vi "2012_01_03 Crunch.vi"(6 "Temp On":dbl, 7 "Motor #":i32, 8 "error in (no error)":errorcluster, 9 "data":waveform(dbl)[](array[waveform]), 10 "Elapsed Time (h)":dbl, 11 "Motor In":T1 {"Elec Power In (W)" format="%.3g"; "Efficiency" format="%#_3g%%"; "Mech Pwr Out (W)" format="%.3g"; "Torque (mNm)" format="%.3g"; "Elapsed Time (h)" format="%.1f"; "Supply (V)" format="%.2f"; "RPM" scale=0.0..40000.0 scale format="%#_4p"}) -> (0 "error out":errorcluster, 2 "Dynamic Data Type":dynamicdata(waveform), 3 "Motor Out":T1={"Enabled"=FALSE, "Fail"=FALSE, "RPM"=0.0, "Motor"=enum."Maxon EC6 6V", "ESC"=enum."Phoenix", "Supply (V)"=0.0, "Test ID and Serial #"="", "Comments"="", "Elapsed Time (h)"=0.0, "Counter"=0.0, "Torque (mNm)"=0.0, "Mech Pwr Out (W)"=0.0, "Efficiency"=0.0, "Elec Power In (W)"=0.0} {"Elec Power In (W)" format="%.3g"; "Efficiency" format="%#_3g%%"; "Mech Pwr Out (W)" format="%.3g"; "Torque (mNm)" format="%.3g"; "Elapsed Time (h)" format="%.1f"; "Supply (V)" format="%.2f"; "RPM" scale=0.0..40000.0 scale format="%#_4p"})   [LabVIEW 2013]
uses:
  MotorTypeDef.ctl
  <vilib>/measure/madcrms.llb/Basic Averaged DC-RMS for 1 Chan.vi
  <vilib>/measure/matone.llb/Extract Single Tone Information 1 Chan.vi
  <vilib>/express/express arith-compare/Formula/XNode/ExpressFormulaBlockNode.xnode
  <vilib>/measure/NI_MAPro.lvlib
panel:
  # "Enable"
  # "Fail"
  # "Enable"
  # "Fail"
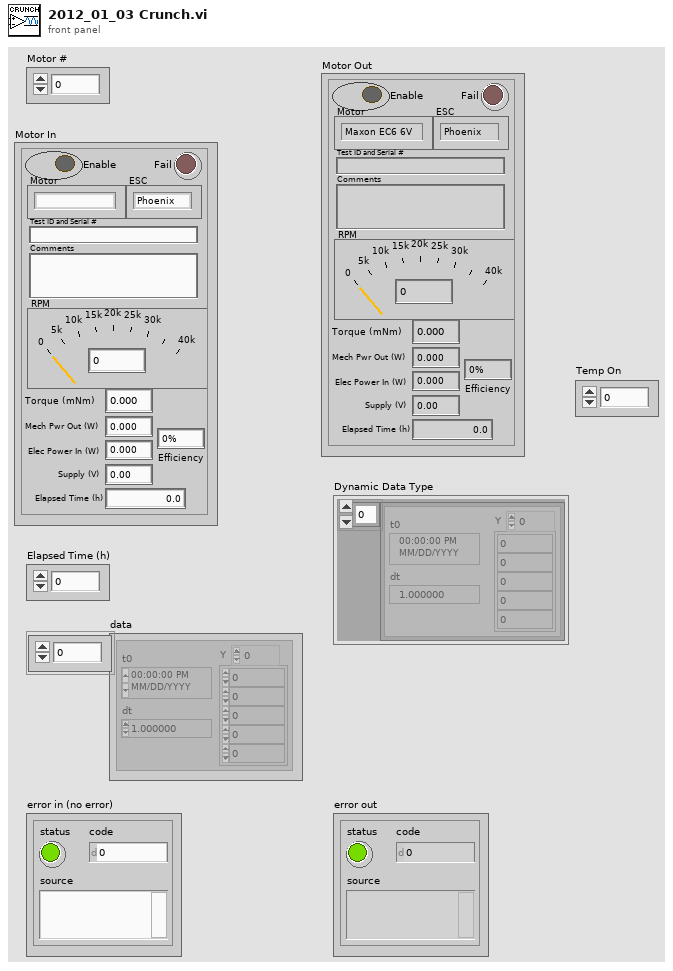
[diagram p1: front panel]
types:
  T1 = typedef "MotorTypeDef.ctl" = cluster{"Enabled":bool, "Fail":bool, "RPM":dbl, "Motor":enum16{"", "Maxon EC6 6V", "Maxon EC4 6V", "FH 0620 6V", "FH 0620 12V"}, "ESC":enum16{"Phoenix", "Maxon", "FH 1801"}, "Supply (V)":dbl, "Test ID and Serial #":string, "Comments":string, "Elapsed Time (h)":dbl, "Counter":dbl, "Torque (mNm)":dbl, "Mech Pwr Out (W)":dbl, "Efficiency":dbl, "Elec Power In (W)":dbl}
  T2 = enum16{"", "Maxon EC6 6V", "Maxon EC4 6V", "FH 0620 6V", "FH 0620 12V"}
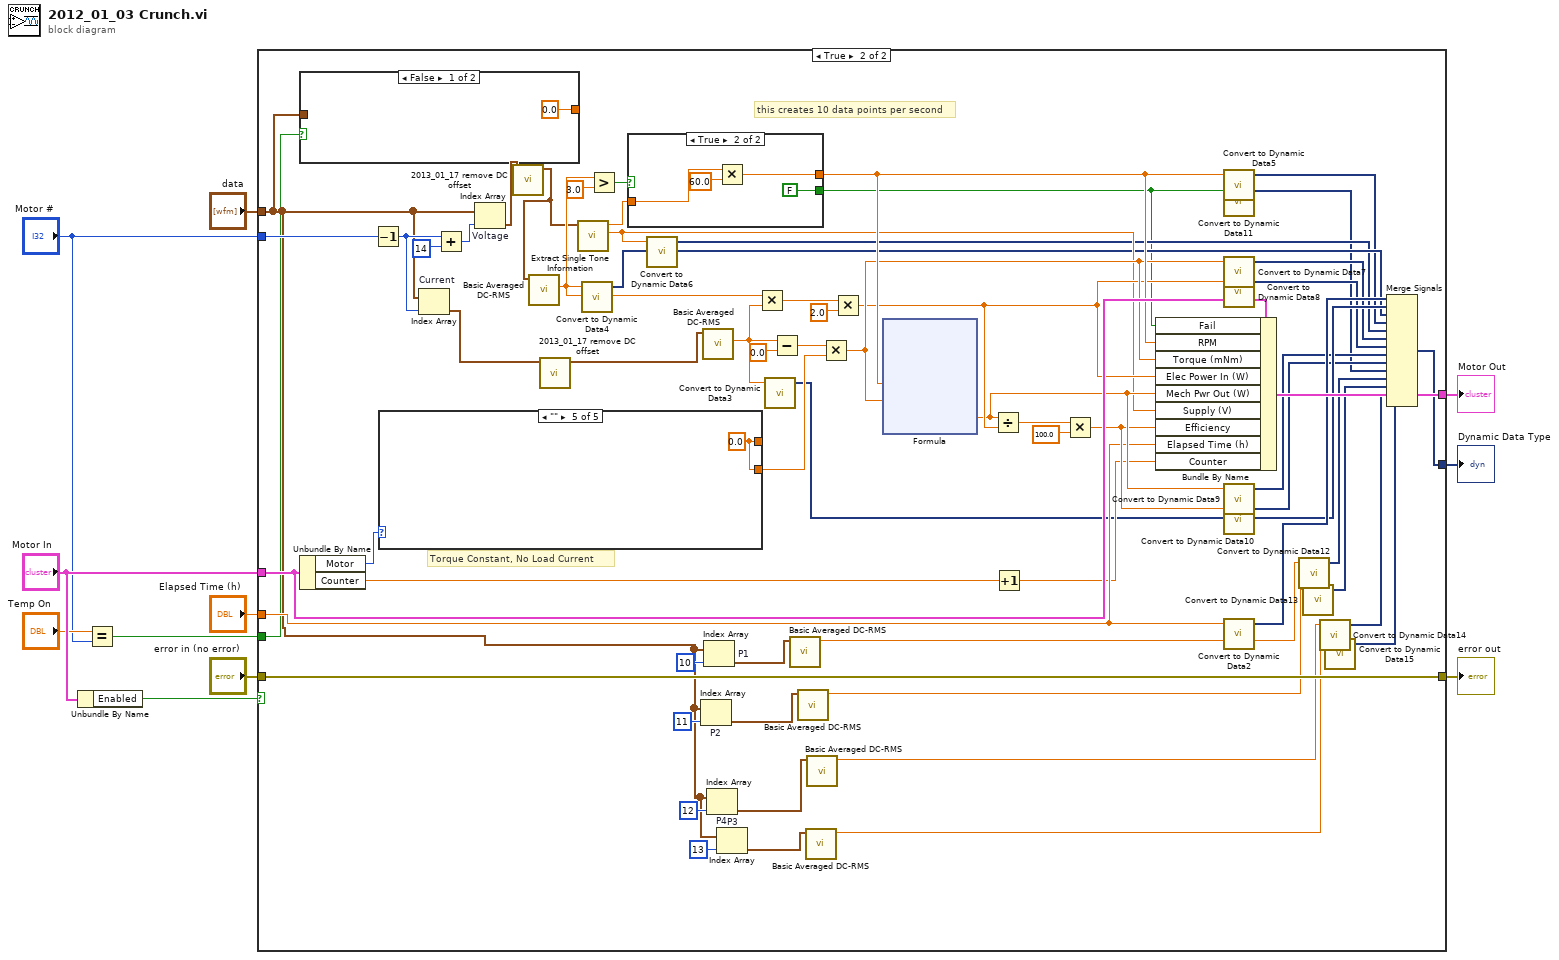
[diagram p0: block diagram]
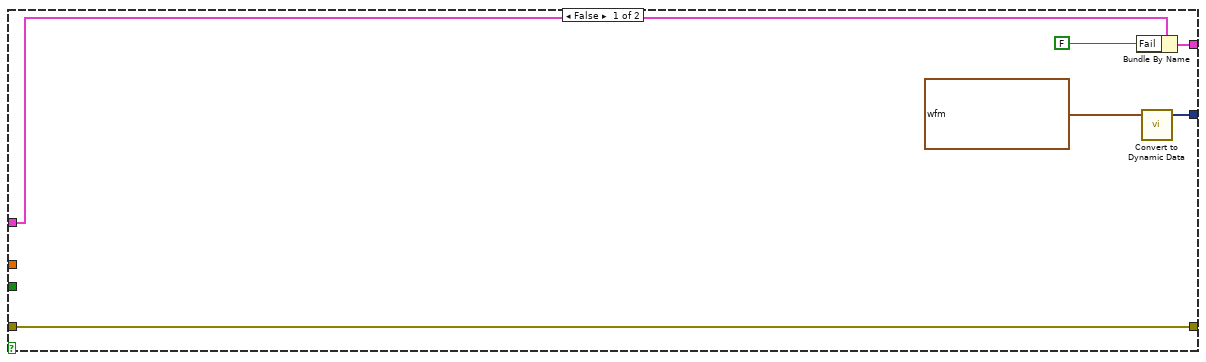
[diagram p2: hidden frame]
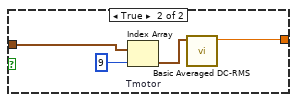
[diagram p3: hidden frame]
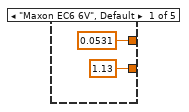
[diagram p4: hidden frame]
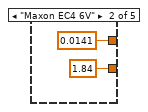
[diagram p5: hidden frame]
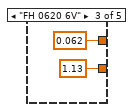
[diagram p6: hidden frame]
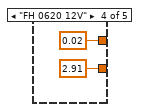
[diagram p7: hidden frame]
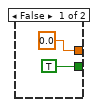
[diagram p8: hidden frame]
diagram:
  n1 = Unbundle By Name("Motor In") -> ("Enabled"=w11:bool)
  n2 = Equal?(x="Temp On", y="Motor #") -> (x = y?=w2:bool)
  n3 = case shown="True" w11 {
    tunnel: "Motor #" -> [_ w65]
    tunnel: "Motor In" -> [w17 w73]
    tunnel: [w16 w72] -> w4
    tunnel: "data" -> [_ w26]
    tunnel: "error in (no error)" -> [w14 w67]
    tunnel: [w14 w67] -> w7
    tunnel: "Elapsed Time (h)" -> [_ w56]
    tunnel: [w12 w44] -> w9
    tunnel: w2 -> [_ w42]
    frame False {
      n4 = Bundle By Name(cluster=w17, "Fail"=FALSE) -> (w16:T1)
      n5 = call "Convert to Dynamic Data"("Waveform"=waveform(dbl) {"t0"=timestamp(0 s since 1904-01-01), "dt"=1.0, "Y"=[]}) -> ("Dynamic Data Type"=w12:dynamicdata)  [unwired: 3 in]
    }
    frame True {
      # "this creates 10 data points per second"
      # "Torque Constant, No Load Current"
      n6 = case shown="False" w42 {
        tunnel: w26 -> [_ w85]
        tunnel: [0.0 ("DC value") w82] -> _
        frame False {
        }
        frame True {
          n7 = Index Array "Tmotor"(array=w85, index=9) -> (element=w83:waveform(dbl))
          n8 = call-poly <vilib>:"Basic Averaged DC-RMS.vi"("signal in"=w83) -> ("DC value"=w82:dbl)  [unwired: 7 in, 3 out]
        }
      }
      n9 = Unbundle By Name(w73) -> ("Motor"=w75:T2, "Counter"=w66:dbl)
      n10 = Decrement(x=w65) -> (x-1=w64:i32)
      n11 = case shown="\"\"" w75 {
        tunnel: [1.13 1.84 1.13 2.91 w104] -> w74
        tunnel: [0.0531 0.0141 0.062 0.02 w104] -> _
        frame "Maxon EC6 6V", Default {
        }
        frame "Maxon EC4 6V" {
        }
        frame "FH 0620 6V" {
        }
        frame "FH 0620 12V" {
        }
        frame "" {
          w104 = 0.0
        }
      }
      n12 = Index Array "Current"(array=w26, index=w64) -> (element=w36:waveform(dbl))
      n13 = Add(x=w64, y=14) -> (x+y=w77:i32)
      n14 = Index Array "Voltage"(array=w26, index=w77) -> (element=w34:waveform(dbl))
      n15 = call "2013_01_17 remove DC offset.vi"("Waveform in"=w34) -> ("Waveform out"=w33:waveform(dbl))  [unwired: 10 in]
      n16 = call-poly <vilib>:"Basic Averaged DC-RMS.vi"("signal in"=w33) -> ("RMS value"=w63:dbl)  [unwired: 7 in, 3 out]
      n17 = call "2013_01_17 remove DC offset.vi"("Waveform in"=w36) -> ("Waveform out"=w35:waveform(dbl))  [unwired: 10 in]
      n18 = call-poly <vilib>:"Extract Single Tone Information.vi"("time signal in"=w33) -> ("detected amplitude"=w58:dbl, "detected frequency"=w76:dbl)  [unwired: 5 in, 4 out]
      n19 = call "Convert to Dynamic Data4"("Double"=w63) -> ("Dynamic Data Type"=w52:dynamicdata)  [unwired: 3 in]
      n20 = Greater?(x=w63, y=3.0) -> (0:w80:bool)
      n21 = case shown="True" w80 {
        tunnel: [0.0 ("y") w110] -> w62
        tunnel: w76 -> [_ w108]
        tunnel: [TRUE FALSE] -> w43
        frame False {
        }
        frame True {
          n22 = Multiply(x=w108, y=60.0) -> (x*y=w110:dbl)
        }
      }
      n23 = call "Convert to Dynamic Data6"("Double"=w58) -> ("Dynamic Data Type"=w50:dynamicdata)  [unwired: 3 in]
      n24 = Index Array "P2"(array=w26, index=11) -> (element=w23:waveform(dbl))
      n25 = call-poly <vilib>:"Basic Averaged DC-RMS.vi"("signal in"=w35) -> ("RMS value"=w39:dbl)  [unwired: 7 in, 3 out]
      n26 = Index Array "P1"(array=w26, index=10) -> (element=w22:waveform(dbl))
      n27 = Index Array "P3"(array=w26, index=12) -> (element=w24:waveform(dbl))
      n28 = Index Array "P4"(array=w26, index=13) -> (element=w25:waveform(dbl))
      n29 = Multiply(x=w63, y=w39) -> (x*y=w71:dbl)
      n30 = call "Convert to Dynamic Data3"("Double"=w39) -> ("Dynamic Data Type"=w53:dynamicdata)  [unwired: 3 in]
      n31 = Subtract(x=w39, y=0.0) -> (x-y=w38:dbl)
      n32 = call-poly <vilib>:"Basic Averaged DC-RMS.vi"("signal in"=w22) -> ("DC value"=w21:dbl)  [unwired: 7 in, 3 out]
      n33 = call-poly <vilib>:"Basic Averaged DC-RMS.vi"("signal in"=w23) -> ("DC value"=w20:dbl)  [unwired: 7 in, 3 out]
      n34 = call-poly <vilib>:"Basic Averaged DC-RMS.vi"("signal in"=w25) -> ("DC value"=w18:dbl)  [unwired: 7 in, 3 out]
      n35 = call-poly <vilib>:"Basic Averaged DC-RMS.vi"("signal in"=w24) -> ("DC value"=w19:dbl)  [unwired: 7 in, 3 out]
      n36 = Multiply(x=w38, y=w74) -> (x*y=w61:dbl)
      n37 = Multiply(x=w71, y=2.0) -> (x*y=w60:dbl)
      n38 = xnode "Formula"("RPM"=w62, "Torque"=w61) -> ("Result"=w59:dbl)  [unwired: 1 in, 1 out]
      n39 = Divide(x=w59, y=w60) -> (x/y=w69:dbl)
      n40 = Increment(x=w66) -> (x+1=w55:dbl)
      n41 = Multiply(x=w69, y=100.0) -> (x*y=w57:dbl)
      n42 = Bundle By Name(cluster=w73, "Fail"=w43, "RPM"=w62, "Torque (mNm)"=w61, "Elec Power In (W)"=w60, "Mech Pwr Out (W)"=w59, "Supply (V)"=w58, "Efficiency"=w57, "Elapsed Time (h)"=w56, "Counter"=w55) -> (w72:T1)
      n43 = call "Convert to Dynamic Data5"("Double"=w62) -> ("Dynamic Data Type"=w51:dynamicdata)  [unwired: 3 in]
      n44 = call "Convert to Dynamic Data11"("Boolean"=w43) -> ("Dynamic Data Type"=w45:dynamicdata)  [unwired: 3 in]
      n45 = call "Convert to Dynamic Data7"("Double"=w61) -> ("Dynamic Data Type"=w49:dynamicdata)  [unwired: 3 in]
      n46 = call "Convert to Dynamic Data8"("Double"=w60) -> ("Dynamic Data Type"=w48:dynamicdata)  [unwired: 3 in]
      n47 = call "Convert to Dynamic Data9"("Double"=w59) -> ("Dynamic Data Type"=w47:dynamicdata)  [unwired: 3 in]
      n48 = call "Convert to Dynamic Data10"("Double"=w57) -> ("Dynamic Data Type"=w46:dynamicdata)  [unwired: 3 in]
      n49 = call "Convert to Dynamic Data2"("Double"=w56) -> ("Dynamic Data Type"=w54:dynamicdata)  [unwired: 3 in]
      n50 = call "Convert to Dynamic Data12"("Double"=w21) -> ("Dynamic Data Type"=w41:dynamicdata)  [unwired: 3 in]
      n51 = call "Convert to Dynamic Data13"("Double"=w20) -> ("Dynamic Data Type"=w40:dynamicdata)  [unwired: 3 in]
      n52 = call "Convert to Dynamic Data14"("Double"=w19) -> ("Dynamic Data Type"=w32:dynamicdata)  [unwired: 3 in]
      n53 = call "Convert to Dynamic Data15"("Double"=w18) -> ("Dynamic Data Type"=w31:dynamicdata)  [unwired: 3 in]
      n54 = Merge Signals(w54, w53, w52, w51, w50, w49, w48, w47, w46, w45, w41, w40, w32, w31) -> (w44:dynamicdata)
    }
  }
  "Dynamic Data Type" <- w9
  "error out" <- w7
  "Motor Out" <- w4
